vi "gfitsio-insert-col.vi"(4 "tunits":string, 6 "tform":string, 7 "ttype":string, 8 "error in (no error)":errorcluster, 10 "insertion point (0:1st column)":i32, 11 "gfits refnum":T1) -> (0 "error out":errorcluster, 3 "dup gfits refnum":T1)   [LabVIEW 2022 SP3, in "gfitsio.lvlib"]
doc: "Insert a column in an ASCII or binary table. When inserting, <B>insertion point</B> specifies the column number that the new column should occupy in the table. Any existing columns from this position and higher are shifted over to allow room for the new column(s). The index number on all the following keywords will be incremented or decremented if necessary to reflect the new position of the column(s) in the table: TBCOLn, TFORMn, TTYPEn, TUNITn, TNULLn, TSCALn, TZEROn, TDISPn, TDIMn, TLMINn, TLMAXn, TDMINn, TDMAXn, TCTYPn, TCRPXn, TCRVLn, TCDLTn, TCROTn, and TCUNIn.\n\nThe FITS Standard recommends that only letters, digits, and the underscore character be used in column names (the ttype parameter) with no embedded spaces. Trailing blank characters are not significant. It is recommended that all the column names in a given table be unique within the first 8 characters, and strongly recommended that the names be unique within the first 16 characters."
uses:
  gfitsio.lvlib
  gfitsio-refnum.ctl
  gfitsio.dll
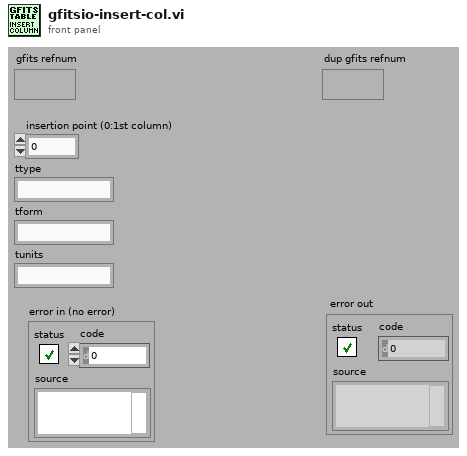
[diagram p1: front panel]
types:
  T1 = typedef "gfitsio.lvlib/gfitsio-refnum.ctl" = refnum<k1>
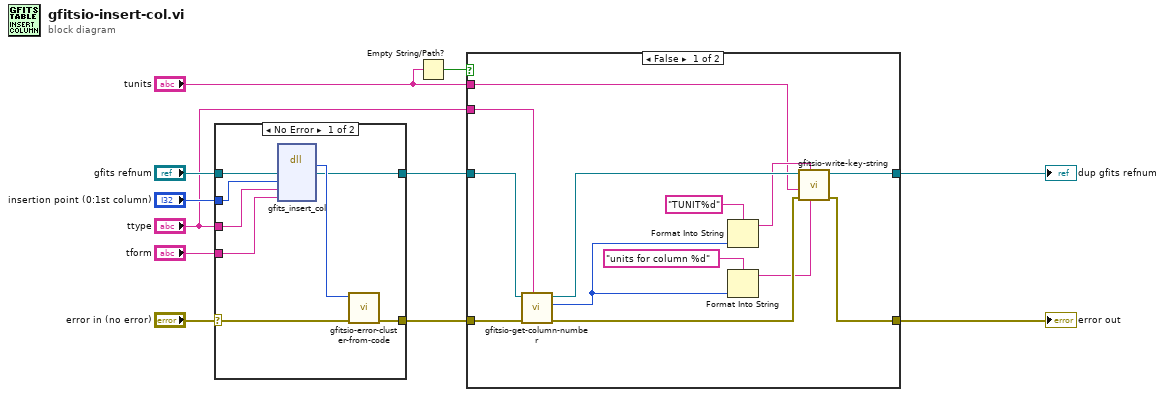
[diagram p0: block diagram]
diagram:
  n1 = case shown="No Error" "error in (no error)" {
    selector: "error in (no error)" -> [w17 w21]
    tunnel: [w19 w21] -> w4
    tunnel: "ttype" -> [w16 _]
    tunnel: "gfits refnum" -> [w14 w20]
    tunnel: [w15 w20] -> w5
    tunnel: "tform" -> [w13 _]
    tunnel: "insertion point (0:1st column)" -> [w12 _]
    frame No Error {
      n2 = dll-call lib="gfitsio.dll" fn="gfits_insert_col"("refnum"=w14, "colnum"=w12, "ttype"=w16, "tform"=w13) -> ("return type"=w18:i32, "refnum"=w15:T1)  [unwired: 6 in, 2 out]
      n3 = call "gfitsio-error-cluster-from-code.vi"("error in (no error)"=w17, "error code"=w18) -> ("error out"=w19:errorcluster)  [unwired: 9 out]
    }
    frame Error {
    }
  }
  n4 = Empty String/Path?(string/path="tunits") -> (empty?=w1:bool)
  n5 = case shown="False" w1 {
    tunnel: [w34 w35] -> w7
    tunnel: [w33 w36] -> w6
    tunnel: w5 -> [w30 w36]
    tunnel: w4 -> [w29 w35]
    tunnel: "ttype" -> [w28 _]
    tunnel: "tunits" -> [w26 _]
    frame False {
      n6 = call "gfitsio-get-column-number.vi"("column"=w28, "error in (no error)"=w29, "gfits refnum"=w30) -> ("error out"=w32:errorcluster, "colnum"=w23:i32, "dup gfits refnum"=w31:T1)  [unwired: 6 in]
      n7 = Format Into String(format string="TUNIT%d" ("value"), w23) -> (resulting string=w27:string)  [unwired: 2 in, 1 out]
      n8 = Format Into String(format string="units for column %d" ("value"), w23) -> (resulting string=w25:string)  [unwired: 2 in, 1 out]
      n9 = call "gfitsio-write-key-string.vi"("comment"=w25, "keyname"=w27, "error in (no error)"=w32, "value"=w26, "gfits refnum"=w31) -> ("error out"=w34:errorcluster, "dup gfits refnum"=w33:T1)  [unwired: 5 in]
    }
    frame True {
    }
  }
  "error out" <- w7
  "dup gfits refnum" <- w6
